vi "CameraInit.vi"(1 "错误输入（无错误）":errorcluster) -> (0 "error out":errorcluster)   [LabVIEW 2012]
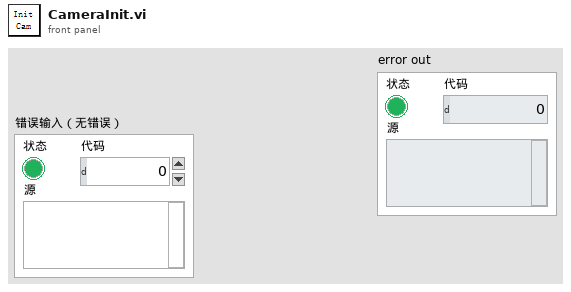
[diagram p1: front panel]
types:
  T1 = typedef "IMAQ Image.ctl" = refnum<image>
  T2 = cluster{"示波器":cluster{"Channel (0:Channel 1)":enum16{"Channel 1", "Channel 2", "Channel 3", "Channel 4"}, "电压范围":dbl, "触发电压":dbl, "时间范围":dbl, " 示波器VISA":refnum<visa-resource-name>}, "光谱仪":cluster{"Channel (0:Channel 1)":enum16{"Channel 1", "Channel 2", "Channel 3", "Channel 4"}, "电压范围":u64, "触发电压":u64, "时间范围":u64}, " 相机1":cluster{"曝光时间":i32, "模拟增益":i32, "控制套接字":i32, "IP 地址":string, " 采集套接字":i32, "  版本号":i32, "ImageData":T1, "  增益最大":i32, "  增益最小":i32, " 曝光最大":i32, " 曝光最小":i32, " 帧速":i32, " 同步切换":i32, "  曝光缩放":i32}, " 偏振仪":cluster{"波长范围":enum16{"可见光", "近红外"}, "电压范围":u64, "触发电压":u64, "时间范围":u64}, " 功率计":cluster{"通道":enum16{"Channel 1", "Channel 2"}, "工作波长":u64, "单位":u64, "时间范围":u64}, "能量计":cluster{"通道":enum16{"Channel 1", "Channel 2"}, "工作波长":u64, "单位":u64, "时间范围":u64}, "电机":cluster{"Channel (0:Channel 1)":enum16{"Channel 1", "Channel 2", "Channel 3", "Channel 4"}, "电压范围":u64, "触发电压":u64, "时间范围":u64}}
  T3 = cluster{"曝光时间":i32, "模拟增益":i32, "控制套接字":i32, "IP 地址":string, " 采集套接字":i32, "  版本号":i32, "ImageData":T1, "  增益最大":i32, "  增益最小":i32, " 曝光最大":i32, " 曝光最小":i32, " 帧速":i32, " 同步切换":i32, "  曝光缩放":i32}
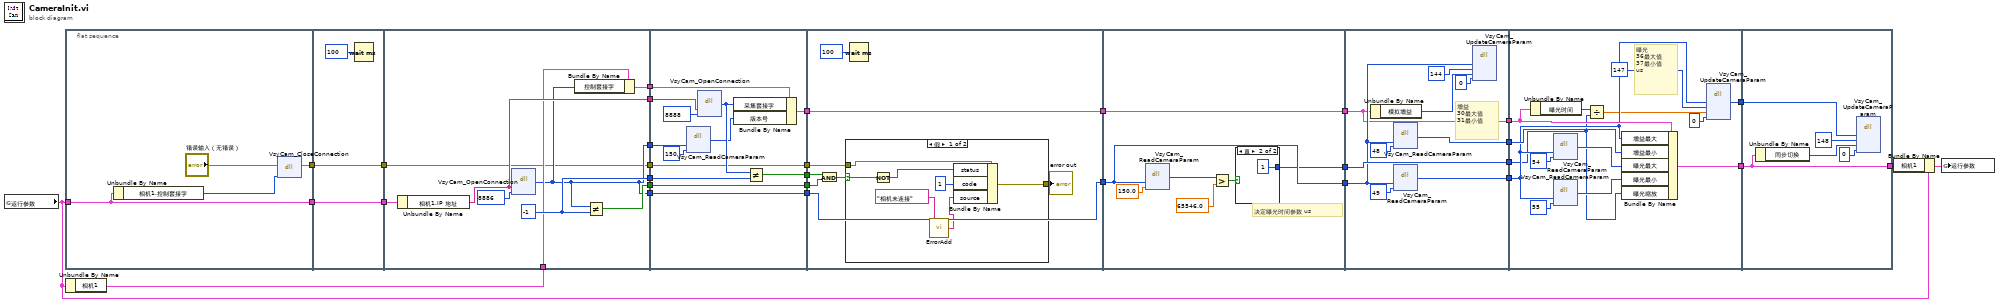
[diagram p0: block diagram]
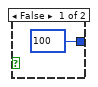
[diagram p3: hidden frame]
diagram:
  n1 = global read "参数.vi" "运行参数"() -> (w6:T2)
  n2 = flat-sequence {
    tunnel: w6 -> [w34]
    tunnel: [w34] -> w31
    tunnel: [w32] -> w1
    tunnel: w31 -> [w37]
    tunnel: [w37] -> w30
    tunnel: [w36] -> w2
    tunnel: w1 -> [w36]
    tunnel: [w46] -> w29
    tunnel: [w45] -> w28
    tunnel: [w41] -> w27
    tunnel: [w41] -> w26
    tunnel: w30 -> [w44]
    tunnel: [w43] -> w25
    tunnel: w8 -> [w42]
    tunnel: [w40] -> w24
    tunnel: [w39] -> w3
    tunnel: w2 -> [w39]
    tunnel: w29 -> [w59]
    tunnel: [w58] -> w23
    tunnel: w28 -> [w58]
    tunnel: [w57] -> w22
    tunnel: [w56] -> w21
    tunnel: w27 -> [w56]
    tunnel: w26 -> [w55]
    tunnel: w25 -> [w53]
    tunnel: w24 -> [w52]
    tunnel: [w49] -> w20
    tunnel: [w48] -> w4
    tunnel: w3 -> [w48]
    tunnel: w23 -> [w68]
    tunnel: w22 -> [w67]
    tunnel: w21 -> [w66]
    tunnel: [w66] -> w19
    tunnel: w20 -> [w64]
    tunnel: [w64] -> w18
    tunnel: w4 -> [w62]
    tunnel: w19 -> [w81]
    tunnel: [w81] -> w17
    tunnel: [w80] -> w16
    tunnel: w18 -> [w77]
    tunnel: [w77] -> w15
    tunnel: w17 -> [w92]
    tunnel: w16 -> [w93]
    tunnel: [w93] -> w14
    tunnel: w15 -> [w87]
    tunnel: [w88] -> w13
    tunnel: [w87] -> w12
    tunnel: [w86] -> w11
    tunnel: w14 -> [w96]
    tunnel: w13 -> [w102]
    tunnel: w12 -> [w104]
    tunnel: w11 -> [w107]
    tunnel: [w98] -> w10
    tunnel: [w97] -> w9
    tunnel: w10 -> [w113]
    tunnel: w9 -> [w110]
    tunnel: [w110] -> w7
    frame #0 {
      n3 = Unbundle By Name(w34) -> ("相机1.控制套接字"=w35:i32)
      n4 = dll-call lib="PTH1?abs D做的项目航天测量软件相机\nVsyCam.dll" fn="VsyCam_CloseConnection"(error in="错误输入（无错误）", "sockFd"=w35) -> (error out=w32:errorcluster)  [unwired: 4 in, 1 out]
    }
    frame #1 {
      n5 = Wait (ms)(milliseconds to wait=u32 100 ("等待时间（毫秒）")) -> ()  [unwired: 1 out]
    }
    frame #2 {
      w46 = -1
      n6 = Unbundle By Name(w44) -> ("相机1.IP 地址"=w43:string)
      n7 = dll-call lib="PTH1?abs D做的项目航天测量软件相机\nVsyCam.dll" fn="VsyCam_OpenConnection"("ip"=w43, "port"=8886) -> ("返回类型"=w41:i32)  [unwired: 5 in, 2 out]
      n8 = Bundle By Name(cluster=w42, "控制套接字"=w41) -> (w40:T3)
      n9 = Not Equal?(x=w41, y=w46) -> (x != y?=w45:bool)
    }
    frame #3 {
      n10 = dll-call lib="PTH1?abs D做的项目航天测量软件相机\nVsyCam.dll" fn="VsyCam_ReadCameraParam"("sockFd"=w55, "cmd"=150) -> ("返回类型"=w50:i32)  [unwired: 5 in, 2 out]
      n11 = dll-call lib="PTH1?abs D做的项目航天测量软件相机\nVsyCam.dll" fn="VsyCam_OpenConnection"("ip"=w53, "port"=8888) -> ("返回类型"=w51:i32)  [unwired: 5 in, 2 out]
      n12 = Bundle By Name(cluster=w52, "采集套接字"=w51, "版本号"=w50) -> (w49:T3)
      n13 = Not Equal?(x=w51, y=w59) -> (x != y?=w57:bool)
    }
    frame #4 {
      n14 = And(x=w67, y=w68) -> (x .and. y?=w63:bool)
      n15 = case shown="假" w63 {
        selector: w63 -> [w74 _]
        tunnel: w62 -> [w75 w76]
        tunnel: [w71 w76] -> w61
        frame False {
          n16 = Not(x=w74) -> (.not. x?=w73:bool)
          n17 = call "ErrorAdd.vi"("source"="相机未连接") -> ("Errorout Souce"=w69:string)
          n18 = Bundle By Name(cluster=w75, "status"=w73, "code"=1, "source"=w69) -> (w71:errorcluster)
        }
        frame True {
        }
      }
      "error out" <- w61
      n19 = Wait (ms)(milliseconds to wait=u32 100 ("等待时间（毫秒）")) -> ()  [unwired: 1 out]
    }
    frame #5 {
      # "决定曝光时间参数 us"
      n20 = dll-call lib="PTH1?abs D做的项目航天测量软件相机\nVsyCam.dll" fn="VsyCam_ReadCameraParam"("sockFd"=w81, "cmd"=150.0) -> ("返回类型"=w78:i32)  [unwired: 5 in, 2 out]
      n21 = Greater?(x=w78, y=65546.0) -> (0:w79:bool)
      n22 = case shown="真" w79 {
        tunnel: [100 1] -> w80
        frame False {
        }
        frame True {
        }
      }
    }
    frame #6 {
      # "增益\n30最大值\n31最小值"
      n23 = Unbundle By Name(w87) -> ("模拟增益"=w89:i32)
      n24 = dll-call lib="PTH1?abs D做的项目航天测量软件相机\nVsyCam.dll" fn="VsyCam_ReadCameraParam"("sockFd"=w92, "cmd"=48) -> ("返回类型"=w86:i32)  [unwired: 5 in, 2 out]
      n25 = dll-call lib="PTH1?abs D做的项目航天测量软件相机\nVsyCam.dll" fn="VsyCam_ReadCameraParam"("sockFd"=w92, "cmd"=49) -> ("返回类型"=w88:i32)  [unwired: 5 in, 2 out]
      n26 = dll-call lib="PTH1?abs D做的项目航天测量软件相机\nVsyCam.dll" fn="VsyCam_UpdateCameraParam"("sockFd"=w92, "command"=144, "value"=w89, "ack"=0) -> ()  [unwired: 8 in, 2 out]
    }
    frame #7 {
      # "曝光\n36最大值\n37最小值\nus"
      n27 = Unbundle By Name(w104) -> ("曝光时间"=w103:i32)
      n28 = dll-call lib="PTH1?abs D做的项目航天测量软件相机\nVsyCam.dll" fn="VsyCam_ReadCameraParam"("sockFd"=w102, "cmd"=54) -> ("返回类型"=w106:i32)  [unwired: 5 in, 2 out]
      n29 = dll-call lib="PTH1?abs D做的项目航天测量软件相机\nVsyCam.dll" fn="VsyCam_ReadCameraParam"("sockFd"=w102, "cmd"=55) -> ("返回类型"=w105:i32)  [unwired: 5 in, 2 out]
      n30 = Divide(x=w103, y=w96) -> (x/y=w100:dbl)
      n31 = Bundle By Name(cluster=w104, "增益最大"=w102, "增益最小"=w107, "曝光最大"=w106, "曝光最小"=w105, "曝光缩放"=w96) -> (w97:T3)
      n32 = dll-call lib="PTH1?abs D做的项目航天测量软件相机\nVsyCam.dll" fn="VsyCam_UpdateCameraParam"("sockFd"=w102, "command"=147, "value"=w100, "ack"=0) -> ("sockFd"=w98:i32)  [unwired: 7 in, 2 out]
    }
    frame #8 {
      n33 = Unbundle By Name(w110) -> ("同步切换"=w112:i32)
      n34 = dll-call lib="PTH1?abs D做的项目航天测量软件相机\nVsyCam.dll" fn="VsyCam_UpdateCameraParam"("sockFd"=w113, "command"=148, "value"=w112, "ack"=0) -> ()  [unwired: 8 in, 2 out]
    }
  }
  n35 = Unbundle By Name(w6) -> ("相机1"=w8:T3)
  n36 = Bundle By Name(cluster=w6, "相机1"=w7) -> (w5:T2)
  n37 = global write "参数.vi" "运行参数"(w5) -> ()
